vi "RemoveDCBG.vi"(9 "Channel":enum16{"DC Only", "Ch1", "Ch2", "Ch3", "Ch4"}(ring), 11 "WF in":dbl[](array[numeric])) -> (1 "Scaled BG":dbl[](array[numeric]), 2 "DC":dbl format="%0.2f", 3 "WF out":dbl[](array[numeric]))   [LabVIEW 2020]
uses:
  <vilib>/Analysis/baseanly.llb/Mean (DBL).vi
  GlobalVariables.vi
  <vilib>/Analysis/NI_AALBase.lvlib
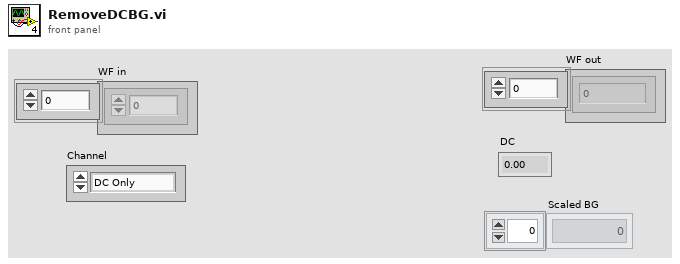
[diagram p1: front panel]
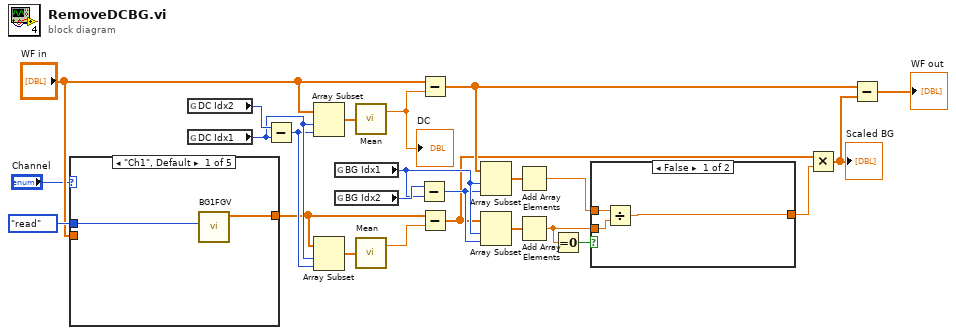
[diagram p0: block diagram]
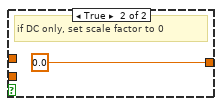
[diagram p2: hidden frame]
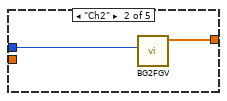
[diagram p3: hidden frame]
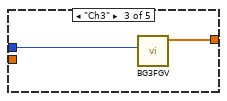
[diagram p4: hidden frame]
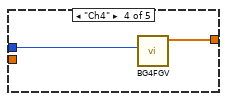
[diagram p5: hidden frame]
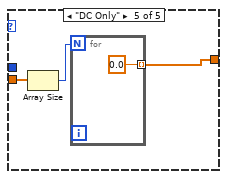
[diagram p6: hidden frame]
diagram:
  n1 = case shown="\"Ch1\", Default" "Channel" {
    tunnel: enum16{"write", "read"}."read" ("action") -> [w26 w28 w30 w32 _]
    tunnel: [w25 w27 w29 w31 w33] -> w14
    tunnel: "WF in" -> [_ _ _ _ w35]
    frame "Ch1", Default {
      n2 = call "BG1FGV.vi"("action"=w26) -> ("BG1 out"=w25:dbl[])  [unwired: 9 in, 1 out]
    }
    frame "Ch2" {
      n3 = call "BG2FGV.vi"("action"=w28) -> ("BG2 out"=w27:dbl[])  [unwired: 9 in, 1 out]
    }
    frame "Ch3" {
      n4 = call "BG3FGV.vi"("action"=w30) -> ("BG3 out"=w29:dbl[])  [unwired: 9 in, 1 out]
    }
    frame "Ch4" {
      n5 = call "BG4FGV.vi"("action"=w32) -> ("BG14out"=w31:dbl[])  [unwired: 9 in, 1 out]
    }
    frame "DC Only" {
      n6 = Array Size(array=w35) -> (size(s)=w34:i32)
      n7 = for {
        N: w34 -> [_]
        tunnel: [0.0] -> w33 mode=indexing
      }
    }
  }
  n8 = global read "GlobalVariables.vi" "DC Idx2"() -> (w22:i32)
  n9 = global read "GlobalVariables.vi" "DC Idx1"() -> (w17:i32)
  n10 = Subtract(x=w22, y=w17) -> (x-y=w16:i32)
  n11 = Array Subset(array="WF in", index=w17, length=w16) -> (w24:dbl[])
  n12 = Array Subset(array=w14, index=w17, length=w16) -> (w15:dbl[])
  n13 = global read "GlobalVariables.vi" "BG Idx1"() -> (w9:i32)
  n14 = global read "GlobalVariables.vi" "BG Idx2"() -> (w20:i32)
  n15 = call-poly <vilib>:"Mean.vi"("X"=w24) -> ("mean"=w23:dbl)  [unwired: 1 out]
  "DC" <- w23
  n16 = call-poly <vilib>:"Mean.vi"("X"=w15) -> ("mean"=w13:dbl)  [unwired: 1 out]
  n17 = Subtract(x=w20, y=w9) -> (x-y=w8:i32)
  n18 = Subtract(x="WF in", y=w23) -> (x-y=w10:dbl[])
  n19 = Subtract(x=w14, y=w13) -> (x-y=w7:dbl[])
  n20 = Array Subset(array=w10, index=w9, length=w8) -> (w11:dbl[])
  n21 = Array Subset(array=w7, index=w9, length=w8) -> (w12:dbl[])
  n22 = Add Array Elements(numeric array=w11) -> (sum=w3:dbl)
  n23 = Add Array Elements(numeric array=w12) -> (sum=w1:dbl)
  n24 = Equal To 0?(x=w1) -> (x = 0?=w4:bool)
  n25 = case shown="False" w4 {
    tunnel: w3 -> [w39 _]
    tunnel: [w38 0.0] -> w2
    tunnel: w1 -> [w37 _]
    frame False {
      n26 = Divide(x=w39, y=w37) -> (x/y=w38:dbl)
    }
    frame True {
      # "if DC only, set scale factor to 0"
    }
  }
  n27 = Multiply(x=w7, y=w2) -> (x*y=w6:dbl[])
  "Scaled BG" <- w6
  n28 = Subtract(x=w10, y=w6) -> (x-y=→"WF out":dbl[])
